vi "genColormap.vi"() -> (3 "Colormap":u32[](array[numeric]))   [LabVIEW 2017]
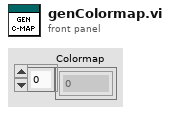
[diagram p1: front panel]
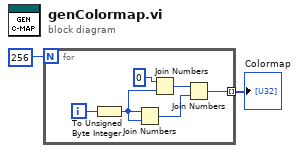
[diagram p0: block diagram]
diagram:
  n1 = for {
    N: 256 -> [_]
    tunnel: [w3] -> w1 mode=indexing
    i -> [w8]
    n2 = To Unsigned Byte Integer(number=w8) -> (unsigned 8bit integer=w6:u8)
    n3 = Join Numbers(hi=w6, lo=w6) -> ((hi.lo)=w5:u16)
    n4 = Join Numbers(hi=u8 0, lo=w6) -> ((hi.lo)=w4:u16)
    n5 = Join Numbers(hi=w4, lo=w5) -> ((hi.lo)=w3:u32)
  }
  "Colormap" <- w1
